vi "Main_SAIDD_v1.1.vi"() -> ()   [LabVIEW 2018]
uses:
  <extravilib>/ChannelInstances/Tag-dbl/Read With Abort.vi
  <extravilib>/ChannelInstances/Tag-bool/Read With Abort.vi
  <extravilib>/ChannelInstances/Tag-u16[State 0 - Default,State 1 - Go down,State 2 - Go up,State 3 - Triangle Wobble]/Read With Abort.vi
  <extravilib>/ChannelInstances/Tag-dbl/Write With Abort.vi
  <extravilib>/ChannelInstances/Tag-bool/Write With Abort.vi
  <extravilib>/ChannelInstances/Tag-u16[State 0 - Default,State 1 - Go down,State 2 - Go up,State 3 - Triangle Wobble]/Write With Abort.vi
  <vilib>/myRIO/Common/Instrument Driver Framework/myRIO v1.0/UART/vis/myRIO v1.0 Close UART.vi
  <vilib>/Utility/error.llb/Error Cluster From Error Code.vi
  <vilib>/myRIO/Common/Instrument Driver Framework/myRIO v1.0/PWM/vis/myRIO v1.0 Write PWM.vi
  <vilib>/myRIO/Common/Instrument Driver Framework/myRIO v1.0/DIO/vis/myRIO v1.0 Write DIO.vi
  <extravilib>/ChannelInstances/Tag-dbl/Instantiate.vi
  <extravilib>/ChannelInstances/Tag-bool/Instantiate.vi
  <extravilib>/ChannelInstances/Tag-u16[State 0 - Default,State 1 - Go down,State 2 - Go up,State 3 - Triangle Wobble]/Instantiate.vi
  <extravilib>/ChannelInstances/Tag-dbl/EndpointRead.vi
  <extravilib>/ChannelInstances/Tag-bool/EndpointRead.vi
  <extravilib>/ChannelInstances/Tag-u16[State 0 - Default,State 1 - Go down,State 2 - Go up,State 3 - Triangle Wobble]/EndpointRead.vi
  <extravilib>/ChannelInstances/Tag-dbl/Endpoint.vi
  <extravilib>/ChannelInstances/Tag-bool/Endpoint.vi
  <extravilib>/ChannelInstances/Tag-u16[State 0 - Default,State 1 - Go down,State 2 - Go up,State 3 - Triangle Wobble]/Endpoint.vi
  <vilib>/myRIO/Common/Instrument Driver Framework/Utilities/vis/FPGA Ref Manager.vi
  <vilib>/myRIO/Common/Instrument Driver Framework/myRIO v1.0/myRIO v1.0 Reset FPGA.vi
  <vilib>/myRIO/Common/Instrument Driver Framework/myRIO v1.0/IRQ/vis/myRIO v1.0 IRQ Info FGV.vi
  <vilib>/myRIO/Common/Instrument Driver Framework/myRIO v1.0/IRQ/vis/myRIO v1.0 Timer IRQ Info FGV.vi
  <vilib>/myRIO/Common/Instrument Driver Framework/myRIO v1.0/IRQ/vis/myRIO v1.0 ISR Agent.vi
  <extravilib>/ChannelInstances/Tag-bool.lvlib
  <vilib>/myRIO/Instrument Drivers/Onboard IO/DIO/DIO.lvlib
  <vilib>/myRIO/Instrument Drivers/Onboard IO/PWM/PWM.lvlib
  <vilib>/myRIO/Instrument Drivers/Utilities/Utilities.lvlib
  <extravilib>/ChannelInstances/Tag-u16[State 0 - Default,State 1 - Go down,State 2 - Go up,State 3 - Triangle Wobble].lvlib
  <extravilib>/ChannelInstances/Tag-dbl.lvlib
panel:
  in  "Tab Control":enum32{"Control", "Test"}(tab)
  in  "Tilt Radius":dbl=0.005 format="%#_13g"
  in  "Cutoff \nFrequency":dbl=900.0
  out "Drill Battery Capacity (%)":dbl(knob) scale=0.0..100.0
  out "Ammeter measurement":dbl(graph)
  in  "Wobble Iterations":i32(knob)=800 scale=500.0..1000.0
  out "Tilt Alarm!":bool
  in  "Stepper \n Frequency":T1(slide)={"Numeric"=120.0, "Numeric"=200.0, "Numeric"=400.0} caption="Stepper Frequency                   Min              Default        Max" scale=100.0..500.0
  in  "Drill Resistance Threshold        Slow            Lower          Upper":T1(slide)={"Numeric"=2750.0, "Numeric"=3025.0, "Numeric"=3100.0} scale=2500.0..3250.0
  out "error out":errorcluster
  in  "Stop":bool
  in  "Enable Triangle Wobble":bool=TRUE
  out "Duty Cycle":dbl
  in  "Drill - Frequency [Hz]":dbl=200.0
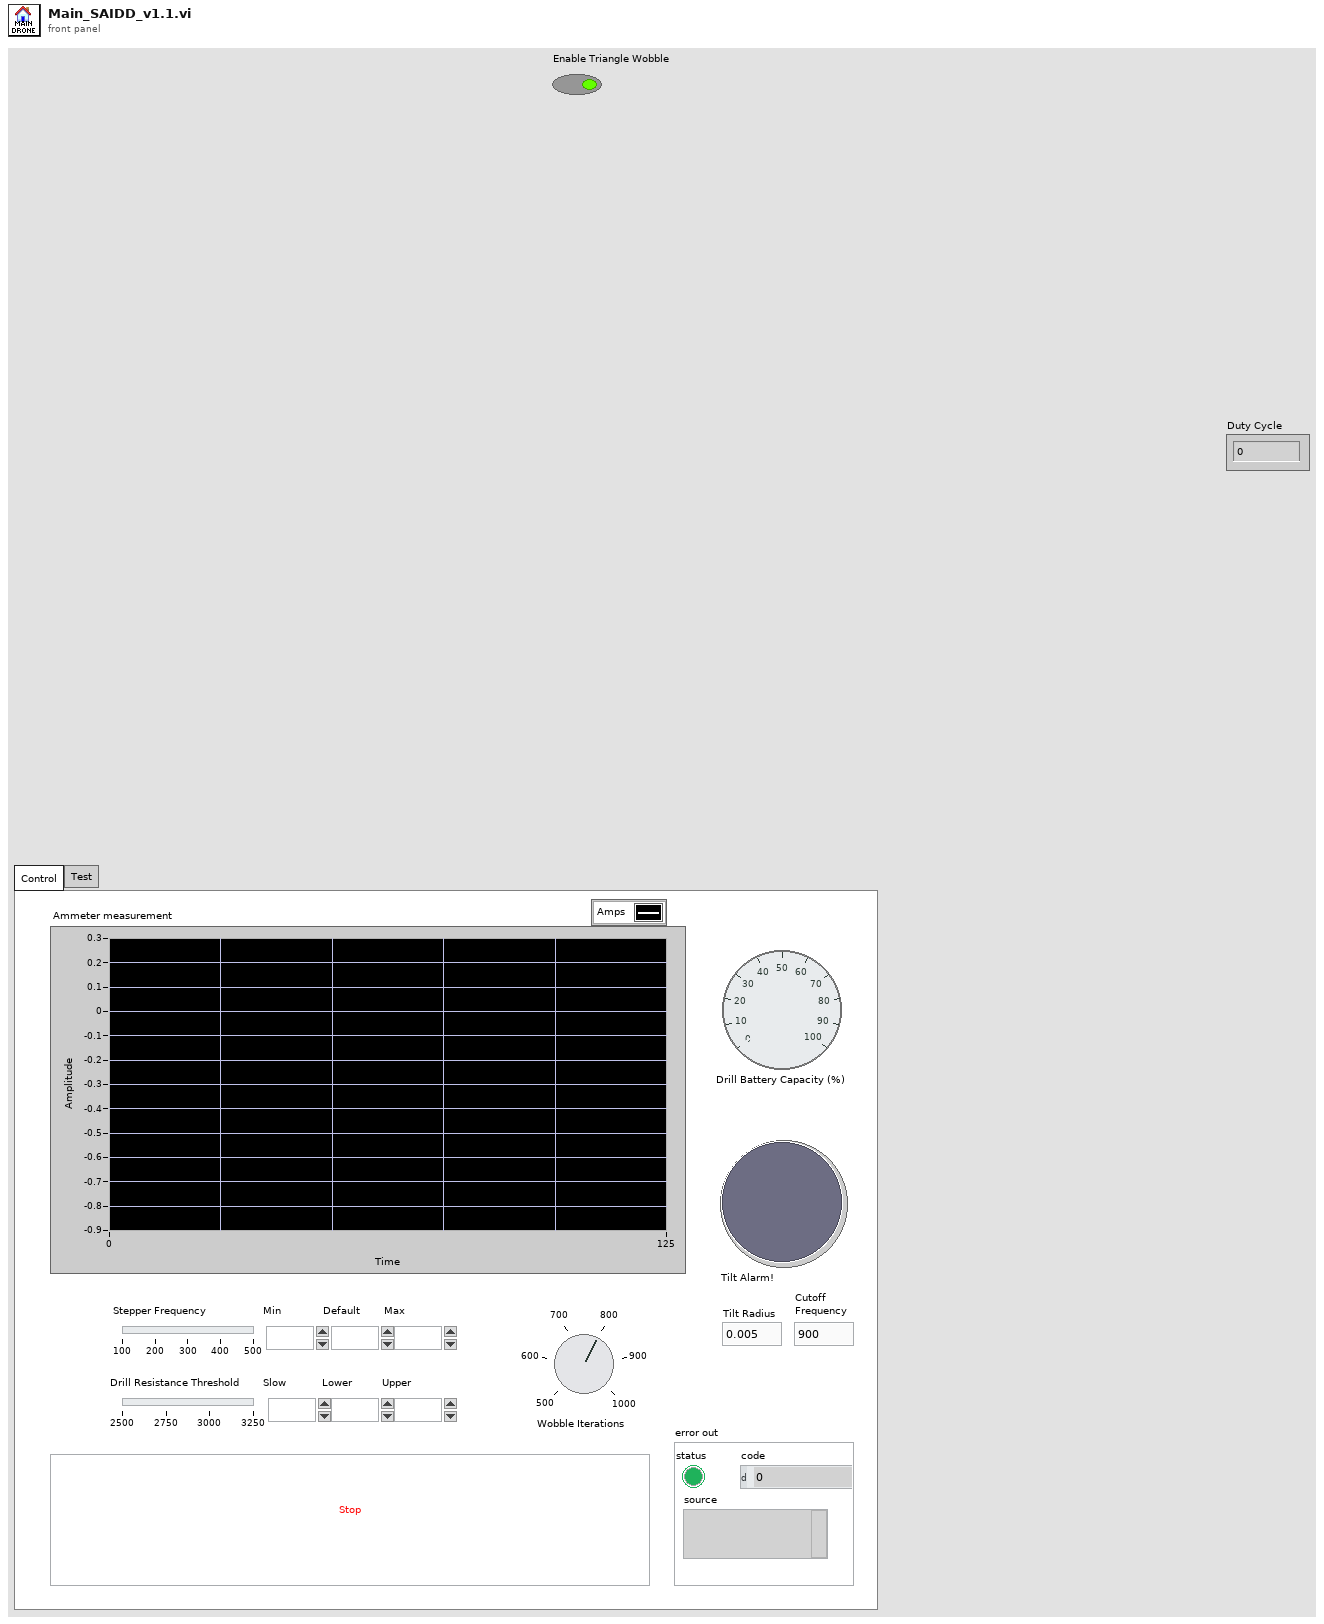
[diagram p1: front panel]
types:
  T1 = cluster{"Numeric":dbl, "Numeric":dbl, "Numeric":dbl}
  T2 = enum16{"State 0 - Default", "State 1 - Go down", "State 2 - Go up", "State 3 - Triangle Wobble"}
  T3 = typedef "DIO.lvlib/DIO Reference.ctl" = cluster{"myRIO Reference":T4, "DIO Channels List":T8}
  T4 = typedef "myRIO Generic Hardware Reference.ctl" = cluster{"myRIO Model":T5, "myRIO Hardware Reference":T6}
  T5 = typedef "Hardware Version Enum.ctl" = enum16{"Unknown", "myRIO-1900", "myRIO-1950", "roboRIO", "NI ELVIS RIO CM", "ELVIS III"}
  T6 = typedef "myRIO v1.0 Reference.ctl" = cluster{"Generic FPGA Reference":T7, "Allow multiple opens":bool}
  T7 = typedef "Generic FPGA Reference.ctl" = refnum<k20>
  T8 = typedef "DIO Channels List.ctl" = T9[]
  T9 = typedef "DIO Channels Enum.ctl" = enum16{"Not Connected", "C/DIO0", "C/DIO1", "C/DIO2", "C/DIO3", "C/DIO4", "C/DIO5", "C/DIO6", "C/DIO7", "A/DIO0", "A/DIO1", "A/DIO2", "A/DIO3", "A/DIO4", "A/DIO5", "A/DIO6", "A/DIO7", "A/DIO8", "A/DIO9", "A/DIO10", "A/DIO11", "A/DIO12", "A/DIO13", "A/DIO14", "A/DIO15", "A/DIO16", "A/DIO17", "A/DIO18", "A/DIO19", "B/DIO0", "B/DIO1", "B/DIO2", "B/DIO3", "B/DIO4", "B/DIO5", "B/DIO6", "B/DIO7", "B/DIO8", "B/DIO9", "B/DIO10", "B/DIO11", "B/DIO12", "B/DIO13", "B/DIO14", "B/DIO15", "B/DIO16", "B/DIO17", "B/DIO18", "B/DIO19", "LED0", "LED1", "LED2", "LED3", "Button0", "DIO/DIO0", "DIO/DIO1", "DIO/DIO2", "DIO/DIO3", "DIO/DIO4", "DIO/DIO5", "DIO/DIO6", "DIO/DIO7", "DIO/DIO8", "DIO/DIO9", "SPI/CS0", "SPI/CS1", "SPI/CS2", "SPI/CS3", "LED RADIO (Green)", "LED RADIO (Red)", "LED COMM (Green)", "LED COMM (Red)", "LED MODE (Green)", "LED MODE (Red)"}
  T10 = typedef "PWM.lvlib/PWM Reference.ctl" = cluster{"myRIO Reference":T4, "PWM Channels Enum":T11, "PWM Configuration":T12}
  T11 = typedef "PWM Channels Enum.ctl" = enum16{"Not Connected", "C/PWM0", "C/PWM1", "A/PWM0", "A/PWM1", "A/PWM2", "A/PWM3", "A/PWM4", "A/PWM5", "A/PWM6", "A/PWM7", "A/PWM8", "A/PWM9", "A/PWM10", "A/PWM11", "A/PWM12", "A/PWM13", "A/PWM14", "A/PWM15", "A/PWM16", "A/PWM17", "A/PWM18", "A/PWM19", "B/PWM0", "B/PWM1", "B/PWM2", "B/PWM3", "B/PWM4", "B/PWM5", "B/PWM6", "B/PWM7", "B/PWM8", "B/PWM9", "B/PWM10", "B/PWM11", "B/PWM12", "B/PWM13", "B/PWM14", "B/PWM15", "B/PWM16", "B/PWM17", "B/PWM18", "B/PWM19", "PWM/PWM0", "PWM/PWM1", "PWM/PWM2", "PWM/PWM3", "PWM/PWM4", "PWM/PWM5", "PWM/PWM6", "PWM/PWM7", "PWM/PWM8", "PWM/PWM9"}
  T12 = typedef "PWM.lvlib/PWM Configuration.ctl" = cluster{"Frequency":dbl, "Duty Cycle":dbl}
  T13 = typedef "Accelerometer.lvlib/Accelerometer Reference.ctl" = cluster{"myRIO Reference":T4, "Accelerometer Channels List":T14, "LSB Weight":dbl}
  T14 = typedef "Accelerometer Channels List.ctl" = T15[]
  T15 = typedef "Accelerometer Channels Enum.ctl" = enum16{"Not Connected", "X-Axis", "Y-Axis", "Z-Axis"}
  T16 = typedef "AI.lvlib/AI Reference.ctl" = cluster{"myRIO Reference":T4, "AI Channels List":T17, "AI Scaling Constants List":T19}
  T17 = typedef "AI Channels List.ctl" = T18[]
  T18 = typedef "AI Channels Enum.ctl" = enum16{"Not Connected", "AudioIn/Left", "AudioIn/Right", "C/AI0", "C/AI1", "A/AI0", "A/AI1", "A/AI2", "A/AI3", "A/AI4", "A/AI5", "A/AI6", "A/AI7", "B/AI0", "B/AI1", "B/AI2", "B/AI3", "B/AI4", "B/AI5", "B/AI6", "B/AI7", "AI/AI0", "AI/AI1", "AI/AI2", "AI/AI3", "A/AI0 (DIFF)", "A/AI1 (DIFF)", "A/AI2 (DIFF)", "A/AI3 (DIFF)", "B/AI0 (DIFF)", "B/AI1 (DIFF)", "B/AI2 (DIFF)", "B/AI3 (DIFF)"}
  T19 = typedef "Analog Scaling Constants List.ctl" = T20[]
  T20 = typedef "Analog Scaling Constants.ctl" = cluster{"LSB Weight (Volts)":dbl, "Offset (Volts)":dbl, "Signed?":bool}
  T21 = typedef "SPI.lvlib/SPI Reference.ctl" = cluster{"myRIO Reference":T4, "SPI Channels Enum":T22, "SPI Configuration":T23}
  T22 = typedef "SPI Channels Enum.ctl" = enum16{"Not Connected", "A/SPI", "B/SPI", "SPI/SPI"}
  T23 = typedef "SPI.lvlib/SPI Configuration.ctl" = cluster{"Frequency [Hz]":dbl, "Clock Phase":T24, "Clock Polarity":T25, "Data Direction":T26, "Frame Length":T27}
  T24 = typedef "SPI Clock Phase.ctl" = enum8{"Leading", "Trailing"}
  T25 = typedef "SPI Clock Polarity.ctl" = enum8{"Low", "High"}
  T26 = typedef "SPI Data Direction.ctl" = enum8{"Most significant bit first", "Least significant bit first"}
  T27 = typedef "SPI Frame Length.ctl" = u8
  T28 = cluster{"B/DIO0 - Stepper Direction":T3, "B/DIO1 - Stepper1 Enable":T3, "B/DIO2 - Stepper2 Enable":T3, "B/DIO3 - Stepper3 Enable":T3, "B/DIO4 - Endstop Stepper1 Top":T3, "B/DIO11 - Endstop Stepper1 Bund":T3, "B/DIO12 - Endstop Stepper2 Top":T3, "B/DIO13 - Endstop Stepper2 Bund":T3, "B/DIO14 - Endstop Stepper3 Top":T3, "B/DIO15 - Endstop Stepper3 Bund":T3, "Deleted - A/DIO0 - Cooler":T3, "A/DIO1 - Beacon drop (dio1)":T3, "A/DIO2 - Beacon drop (dio0)":T3, "A/DIO3 - QuickRelease (dio1)":T3, "A/DIO4 - QuickRelease (dio0)":T3, "Deleted - A/DIO11 - LiDAR SPI CS":T3, "B/PWM0 - Stepper":T10, "B/PWM1 - Drill":T10, "Deleted - A/PWM0 - Servo_Roll":T10, "Deleted - A/PWM1 - Servo_Yaw":T10, "Acc. X-axis":T13, "Acc. Y-axis":T13, "B/AI0 - Drone Grounded S1 - F3":T16, "A/AI0 - QuickRelease S4 - F4":T16, "B/AI2 - Beacon Drop S5 - F5":T16, "B/AI3 - Begin drilling S3 - F6":T16, "B/AI1 - Gimbal Seach S8 - F8":T16, "Deleted - A/AI1 - Beacon Wiper":T16, "A/AI2 - QuickRelease Wiper":T16, "A/AI3 - Drill Current":T16, "Deleted - A/SPI - LiDAR":T21, "B/UART - XBee":refnum<visa-resource-name>, "Deleted - A/UART - A3 GPS":refnum<visa-resource-name>, "RIO Flashing LEDs":T3}
  T29 = typedef "Tag-dbl.lvlib/))Channel.ctl" = refnum<queue>
  T30 = typedef "Tag-bool.lvlib/))Channel.ctl" = refnum<queue>
  T31 = typedef "Tag-u16[State 0 - Default,State 1 - Go down,State 2 - Go up,State 3 - Triangle Wobble].lvlib/))Channel.ctl" = refnum<queue>
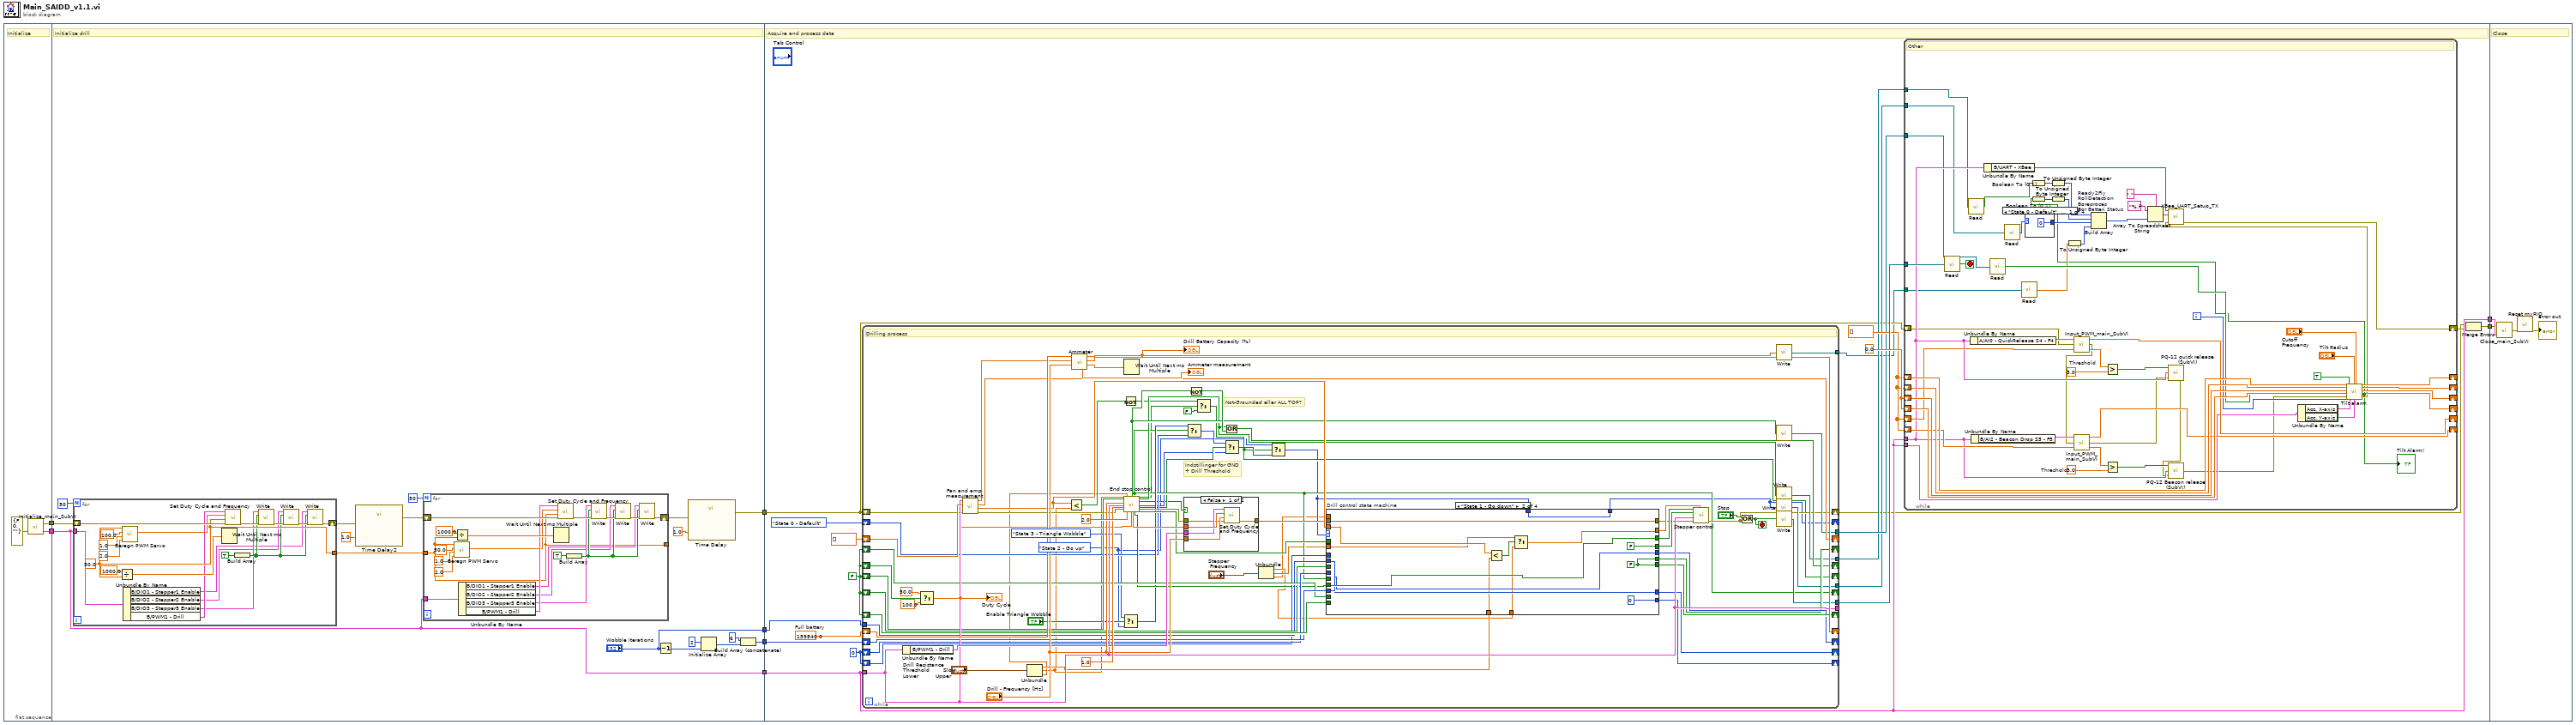
[diagram p0: block diagram]
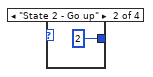
[diagram p2: hidden frame]
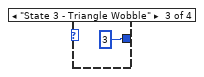
[diagram p3: hidden frame]
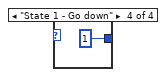
[diagram p4: hidden frame]
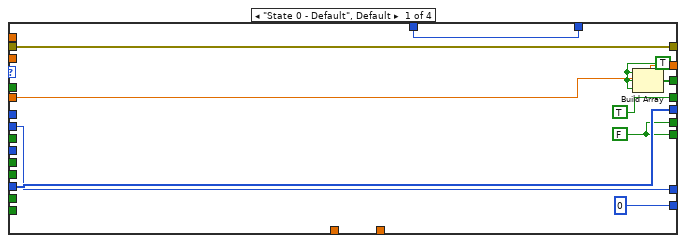
[diagram p6: hidden frame]
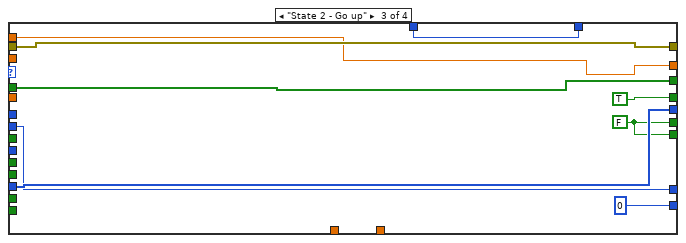
[diagram p7: hidden frame]
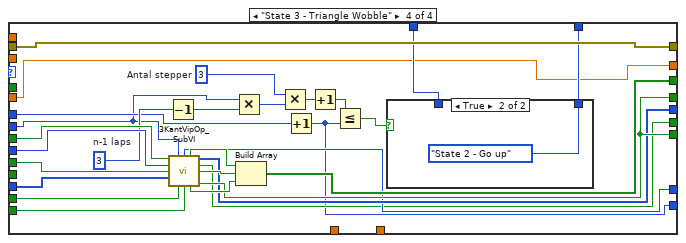
[diagram p8: hidden frame]
diagram:
  n1 = flat-sequence {
    tunnel: [w11] -> w7
    tunnel: [w10] -> w1
    tunnel: w7 -> [w28]
    tunnel: [w28] -> w6
    tunnel: ["Wobble Iterations"] -> w5
    tunnel: [w23] -> w4
    tunnel: [w16] -> w3
    tunnel: w1 -> [w18]
    tunnel: w6 -> [w78]
    tunnel: [w78] -> w8
    tunnel: w5 -> [w81]
    tunnel: w4 -> [w80]
    tunnel: w3 -> [w72]
    tunnel: [w71] -> w2
    tunnel: w8 -> [w299]
    tunnel: w2 -> [w297]
    frame #0 {
      # "Initialize"
      n2 = call "Initialize_main_SubVI.vi"("error in (no error)"=errorcluster {"status"=FALSE, "code"=0, "source"=""}) -> ("output cluster"=w11:T28, "error out"=w10:errorcluster)  [unwired: 1 in]
    }
    frame #1 {
      # "Initialize drill"
      n3 = for {
        N: 50 -> [_]
        tunnel: [w61] -> w21
        shift-right: [w54] -> w19
        shift-left: w18 -> [w63]
        tunnel: w28 -> [w59]
        w61 = 50.0 ("Frequency [Hz]")
        n4 = Divide(x=1000.0, y=w61) -> (x/y=w62:dbl)
        n5 = call "Beregn PWM Servo.vi"("Max (ms puls bredde)"=2.0, "Min (ms puls bredde)"=1.0, "Duty Cycle"=100.0, "Frekvens"=w61) -> ("Output Dutycycle til PWM Servo"=w48:dbl)  [unwired: 7 in]
        n6 = Unbundle By Name(w59) -> ("B/DIO1 - Stepper1 Enable"=w49:T3, "B/DIO2 - Stepper2 Enable"=w50:T3, "B/DIO3 - Stepper3 Enable"=w51:T3, "B/PWM1 - Drill"=w53:T10)
        n7 = Wait Until Next ms Multiple(millisecond multiple=w62) -> ()  [unwired: 1 out]
        n8 = call <vilib>:"Set Duty Cycle and Frequency.vi"("error in (no error)"=w63, "Frequency [Hz]"=w61, "Duty Cycle"=w48, "PWM Ref In"=w53) -> ("error out"=w57:errorcluster)  [unwired: 5 in, 1 out]
        n9 = Build Array(TRUE) -> (w52:bool[])
        n10 = call <extravilib>:"Write.vi"("error in (no error)"=w57, "Values"=w52, "DIO Ref In"=w51) -> ("error out"=w56:errorcluster)  [unwired: 6 in, 1 out]
        n11 = call <extravilib>:"Write.vi"("error in (no error)"=w56, "Values"=w52, "DIO Ref In"=w50) -> ("error out"=w55:errorcluster)  [unwired: 6 in, 1 out]
        n12 = call <extravilib>:"Write.vi"("error in (no error)"=w55, "Values"=w52, "DIO Ref In"=w49) -> ("error out"=w54:errorcluster)  [unwired: 6 in, 1 out]
      }
      n13 = call "Time Delay2"("error in (no error)"=w19, "Delay Time (s)"=1.0) -> ("error out"=w20:errorcluster)  [unwired: 9 in]
      n14 = for {
        N: 50 -> [_]
        tunnel: [w29] -> _
        shift-right: [w36] -> w17
        shift-left: w20 -> [w44]
        tunnel: w28 -> [w41]
        tunnel: w21 -> [w29]
        n15 = call "Beregn PWM Servo.vi"("Max (ms puls bredde)"=2.0, "Min (ms puls bredde)"=1.0, "Duty Cycle"=50.0, "Frekvens"=w29) -> ("Output Dutycycle til PWM Servo"=w30:dbl)  [unwired: 7 in]
        n16 = Divide(x=1000.0, y=w29) -> (x/y=w43:dbl)
        n17 = Unbundle By Name(w41) -> ("B/DIO1 - Stepper1 Enable"=w31:T3, "B/DIO2 - Stepper2 Enable"=w32:T3, "B/DIO3 - Stepper3 Enable"=w33:T3, "B/PWM1 - Drill"=w35:T10)
        n18 = Wait Until Next ms Multiple(millisecond multiple=w43) -> ()  [unwired: 1 out]
        n19 = call <vilib>:"Set Duty Cycle and Frequency.vi"("error in (no error)"=w44, "Frequency [Hz]"=w29, "Duty Cycle"=w30, "PWM Ref In"=w35) -> ("error out"=w39:errorcluster)  [unwired: 5 in, 1 out]
        n20 = Build Array(TRUE) -> (w34:bool[])
        n21 = call <extravilib>:"Write.vi"("error in (no error)"=w39, "Values"=w34, "DIO Ref In"=w33) -> ("error out"=w38:errorcluster)  [unwired: 6 in, 1 out]
        n22 = call <extravilib>:"Write.vi"("error in (no error)"=w38, "Values"=w34, "DIO Ref In"=w32) -> ("error out"=w37:errorcluster)  [unwired: 6 in, 1 out]
        n23 = call <extravilib>:"Write.vi"("error in (no error)"=w37, "Values"=w34, "DIO Ref In"=w31) -> ("error out"=w36:errorcluster)  [unwired: 6 in, 1 out]
      }
      n24 = Decrement(x="Wobble Iterations") -> (x-1=w27:i32)
      n25 = call "Time Delay"("error in (no error)"=w17, "Delay Time (s)"=1.0) -> ("error out"=w16:errorcluster)  [unwired: 9 in]
      n26 = Initialize Array(2, w27) -> (w26:i32[])
      n27 = Build Array (concatenate)(6, w26) -> (w23:i32[])
    }
    frame #2 {
      w82 = 0.0 ("X-Stored-Shift-out")
      w83 = 0 ("Loops shift out")
      w79 = FALSE ("t")
      w85 = 159840.0  # Full battery
      w76 = dbl[] [] ("X-Array-Shift-out")
      # "Acquire and process data"
      n28 = while {
        shift-right: [w175] -> w69
        shift-left: w72 -> [w213]
        shift-right: [w192] -> _
        shift-left: dbl[] [] -> [w224]
        shift-right: [w220] -> _
        shift-left: w85 -> [w221]
        tunnel: w78 -> [w218]
        tunnel: [w218] -> _
        shift-right: [w162] -> _
        shift-left: w79 -> [w214]
        shift-right: [w188] -> _
        shift-left: w79 -> [w211]
        shift-right: [w209] -> _
        shift-left: w79 -> [w208]
        shift-right: [w207] -> _
        shift-left: w80 -> [w206]
        tunnel: w81 -> [w200]
        shift-right: [w204] -> _
        shift-left: w83 -> [w205]
        shift-right: [w203] -> _
        shift-left: w79 -> [w202]
        shift-right: [w173] -> _
        shift-left: w79 -> [w201]
        shift-right: [w198] -> _
        shift-left: w83 -> [w199]
        tunnel: [w185] -> w77
        tunnel: [w183] -> w75
        tunnel: [w182] -> w74
        tunnel: [w180] -> w73
        shift-right: [w157] -> _
        shift-left: T2."State 0 - Default" ("Enum") -> [w172]
        tunnel: [w159] -> w67
        stop <- w186 stop-if-true
        w149 = T2."State 2 - Go up" ("Enum")
        # "Not-Grounded eller ALL TOP?"
        # "Indstillinger for GND \n+ Drill Threshold"
        # "Drilling process"
        n29 = Unbundle By Name(w218) -> ("B/PWM1 - Drill"=w219:T10)
        n30 = Select(t=50.0, s=w211, f=100.0 ("upper limit")) -> (s? t:f=w190:dbl)
        "Duty Cycle" <- w190
        n31 = call "Fan and amp measurement.vi"("error in (no error)"=w213, "Array in"=w224, "output cluster"=w218) -> ("error out"=w179:errorcluster, "Mean out"=w191:dbl, "Array out"=w192:dbl[], "dbl Scaled Value"=w216:dbl)  [unwired: 5 in]
        n32 = Unbundle("Drill Resistance Threshold        Slow            Lower          Upper") -> ("Numeric"=w153:dbl, "Numeric"=w150:dbl, "Numeric"=w152:dbl)
        n33 = Less?(x=w191, y=w150) -> (x < y?=w161:bool)
        n34 = call "Ammeter.vi"("Bor - Frequency [Hz]"="Drill - Frequency [Hz]", "Måling ammeter"=w216, "Sum batteri shift in"=w221) -> ("Wait ud"=w215:dbl, "Sum batteri shift ud"=w220:dbl, "Batteri tilbage (%)"=w160:dbl, "Målt ampere"=→"Ammeter measurement":dbl)  [unwired: 5 in]
        "Drill Battery Capacity (%)" <- w160
        n35 = Not(x=w161) -> (.not. x?=w164:bool)
        n36 = Select(t=T2."State 3 - Triangle Wobble" ("Enum"), s="Enable Triangle Wobble", f=w149) -> (s? t:f=w174:T2)
        n37 = Wait Until Next ms Multiple(millisecond multiple=w215) -> ()  [unwired: 1 out]
        n38 = call "End stop control.vi"("Threshold Lower"=w150, "t"=w214, "Bor - Frequency [Hz]"="Drill - Frequency [Hz]", "output cluster"=w218, "Min (ms puls bredde)"=1.0, "error in (no error)"=w179, "Threshold Upper"=w152, "Max (ms puls bredde)"=2.0, "Bor - Duty Cycle"=w190) -> ("Grounded?"=w184:bool, "Output Dutycycle \nPWM"=w223:dbl, "ALL BOTTOM"=w173:bool, "Bottom Array"=w195:bool[], "Within Drill limits?"=w165:bool, "ALL TOP"=w181:bool, "Move Only?"=w151:bool, "Movement Output"=w168:T2, "HOLD"=w171:bool, "error out"=w178:errorcluster, "Top Array"=w194:bool[])  [unwired: 8 in]
        n39 = case shown="False" w151 {
          tunnel: w223 -> [w231 _]
          tunnel: "Drill - Frequency [Hz]" -> [w230 _]
          tunnel: w219 -> [w229 _]
          tunnel: w178 -> [w228 w232]
          tunnel: [w227 w232] -> w177
          frame False {
            n40 = call <vilib>:"Set Duty Cycle and Frequency.vi"("error in (no error)"=w228, "Frequency [Hz]"=w230, "Duty Cycle"=w231, "PWM Ref In"=w229) -> ("error out"=w227:errorcluster)  [unwired: 5 in, 1 out]
          }
          frame True {
          }
        }
        n41 = Select(t=w174, s=w173, f=w172) -> (s? t:f=w170:T2)
        n42 = Not(x=w184) -> (.not. x?=w187:bool)
        n43 = Select(t=w164, s=w165, f=FALSE) -> (s? t:f=w162:bool)
        n44 = Or(x=w181, y=w187) -> (x .or. y?=w188:bool)
        n45 = Select(t=w170, s=w171, f=w168) -> (s? t:f=w169:T2)
        n46 = Unbundle("Stepper \n Frequency") -> ("Numeric"=w148:dbl, "Numeric"=w155:dbl, "Numeric"=w147:dbl)
        n47 = Select(t=w149, s=w162, f=w169) -> (s? t:f=w158:T2)
        n48 = case "Drill control state machine" shown="\"State 1 - Go down\"" w158 {
          tunnel: [w240 w256 w265 w289] -> w193
          tunnel: w195 -> [_ w256 _ _]
          tunnel: w194 -> [_ _ w265 _]
          tunnel: [TRUE FALSE TRUE w288] -> w217
          tunnel: w177 -> [w239 w254 w263 w293]
          tunnel: [w239 w254 w263 w293] -> w176
          tunnel: [w233 w252 w257 w266] -> w212
          tunnel: w191 -> [_ w251 _ _]
          tunnel: [w236 w248 w260 w288] -> w209
          tunnel: w208 -> [_ _ _ w287]
          tunnel: [w238 w250 w262 w286] -> w207
          tunnel: w206 -> [w238 w250 w262 w285]
          tunnel: w200 -> [w237 w249 w261 w275]
          tunnel: w205 -> [_ _ _ w284]
          tunnel: [w237 w249 w261 w283] -> w204
          tunnel: [w236 w248 w260 w282] -> w203
          tunnel: w202 -> [_ _ _ w281]
          tunnel: w201 -> [_ _ _ w280]
          tunnel: w173 -> [_ _ _ w278]
          tunnel: w199 -> [_ _ _ w277]
          tunnel: [0 0 0 w272] -> w198
          tunnel: w158 -> [w234 w246 w258 w268]
          tunnel: [w234 w246 w258 w267] -> w157
          tunnel: w155 -> [w233 w245 _ w266]
          tunnel: w147 -> [_ _ w257 _]
          tunnel: w148 -> [_ w244 _ _]
          tunnel: w153 -> [_ w243 _ _]
          frame "State 0 - Default", Default {
            w236 = FALSE
            w241 = TRUE
            n49 = Build Array(w241, w241, w241) -> (w240:bool[])
          }
          frame "State 1 - Go down" {
            w248 = FALSE
            n50 = Less?(x=w251, y=w243) -> (x < y?=w253:bool)
            n51 = Select(t=w245, s=w253, f=w244) -> (s? t:f=w252:dbl)
          }
          frame "State 2 - Go up" {
            w260 = FALSE
          }
          frame "State 3 - Triangle Wobble" {
            w273 = 3  # Antal stepper
            w279 = 3  # n-1 laps
            n52 = Decrement(x=w279) -> (x-1=w276:i32)
            n53 = call "3KantVipOp_SubVI.vi"("Shift 1 in"=w280, "Antal iterationer pr. stepper"=w275, "Loops shift in"=w284, "BUND!"=w278, "Index step array shift in"=w285, "Shift 2 in"=w281, "Shift 3 in"=w287) -> ("Loops shift out"=w283:i32, "Enable 1"=w290:bool, "Index step array shift ud"=w286:i32[], "Shift 2 ud"=w282:bool, "Enable 2"=w291:bool, "Enable 3"=w292:bool, "Direction"=w288:bool)  [unwired: 1 in, 1 out]
            n54 = Multiply(x=w275, y=w276) -> (x*y=w274:i32)
            n55 = Build Array(w290, w291, w292) -> (w289:bool[])
            n56 = Multiply(x=w273, y=w274) -> (x*y=w270:i32)
            n57 = Increment(x=w277) -> (x+1=w272:i32)
            n58 = Increment(x=w270) -> (x+1=w269:i32)
            n59 = Less Or Equal?(x=w269, y=w272) -> (x <= y?=w271:bool)
            n60 = case shown="True" w271 {
              tunnel: w268 -> [w294 _]
              tunnel: [w294 T2."State 2 - Go up" ("Enum")] -> w267
              frame False {
              }
              frame True {
              }
            }
          }
        }
        n61 = call "Stepper control.vi"("Stepper frekvens"=w212, "error in (no error)"=w176, "output cluster"=w218, "Direction shift ud"=w217, "Array"=w193) -> ("error out"=w175:errorcluster)  [unwired: 6 in]
        n62 = Or(x="Stop", y=w175) -> (x .or. y?=w186:bool)
        n63 = call <extravilib>:"Write.vi"("element"=w160) -> ("channel"=w159:T29)  [unwired: 1 out]
        n64 = call <extravilib>:"Write.vi"("element"=w184) -> ("channel"=w183:T30)  [unwired: 1 out]
        n65 = call <extravilib>:"Write.vi"("element"=w181) -> ("channel"=w180:T30)  [unwired: 1 out]
        n66 = call <extravilib>:"Write.vi"("element"=w157) -> ("channel"=w182:T31)  [unwired: 1 out]
        n67 = call <extravilib>:"Write.vi"("element"=w186) -> ("channel"=w185:T30)  [unwired: 1 out]
      }
      n68 = while {
        shift-right: [w137] -> _
        shift-left: w76 -> [w142]
        shift-right: [w136] -> _
        shift-left: w76 -> [w141]
        shift-right: [w135] -> _
        shift-left: w82 -> [w140]
        shift-right: [w134] -> _
        shift-left: w82 -> [w139]
        tunnel: w77 -> [w133]
        tunnel: w78 -> [w126]
        tunnel: w78 -> [w127]
        shift-right: [w131] -> _
        shift-left: w76 -> [w130]
        shift-right: [w129] -> _
        shift-left: w76 -> [w128]
        tunnel: w75 -> [w125]
        tunnel: w74 -> [w123]
        tunnel: w73 -> [w122]
        shift-right: [w93] -> w70
        shift-left: w72 -> [w94]
        tunnel: w67 -> [w92]
        i -> [w138]
        stop <- w132 stop-if-true
        w115 = 3.0  # Threshold
        w121 = 3.0  # Threshold
        # "Other"
        n69 = call <extravilib>:"Read.vi"("channel"=w133) -> ("element"=w132:bool)  [unwired: 1 in, 1 out]
        n70 = call <extravilib>:"Read.vi"("channel"=w122) -> ("element"=w96:bool)  [unwired: 1 in, 1 out]
        n71 = Unbundle By Name(w127) -> ("A/AI0 - QuickRelease S4 - F4"=w117:T16)
        n72 = Unbundle By Name(w127) -> ("B/AI2 - Beacon Drop S5 - F5"=w119:T16)
        n73 = Unbundle By Name(w127) -> ("B/UART - XBee"=w107:refnum<visa-resource-name>)
        n74 = call <extravilib>:"Read.vi"("channel"=w125) -> ("element"=w124:bool)  [unwired: 1 in, 1 out]
        n75 = call <extravilib>:"Read.vi"("channel"=w123) -> ("element"=w97:T2)  [unwired: 1 in, 1 out]
        n76 = call <extravilib>:"Read.vi"("channel"=w92) -> ("element"=w90:dbl)  [unwired: 1 in, 1 out]
        n77 = case shown="\"State 0 - Default\", Default" w97 {
          tunnel: [u8 0 u8 2 u8 3 u8 1] -> w102
          frame "State 0 - Default", Default {
          }
          frame "State 2 - Go up" {
          }
          frame "State 3 - Triangle Wobble" {
          }
          frame "State 1 - Go down" {
          }
        }
        n78 = Boolean To (0,1)(Boolean=w96) -> (0, 1=w101:i16)
        n79 = To Unsigned Byte Integer(number=w101) -> (unsigned 8bit integer=w100:u8)
        n80 = To Unsigned Byte Integer(number=w90) -> (unsigned 8bit integer=w91:u8)
        n81 = call "Input_PWM_main_SubVI.vi"("Shift in"=w130, "error in (no error)"=w94, "AI Ref In"=w117) -> ("Value out"=w116:dbl, "error out"=w113:errorcluster, "Shift out"=w131:dbl[])
        n82 = call "Input_PWM_main_SubVI.vi"("Shift in"=w128, "error in (no error)"=w113, "AI Ref In"=w119) -> ("Value out"=w120:dbl, "error out"=w89:errorcluster, "Shift out"=w129:dbl[])
        n83 = Greater?(x=w116, y=w115) -> (0:w114:bool)
        n84 = Greater?(x=w120, y=w121) -> (0:w118:bool)
        n85 = call "PQ-12 quick release (SubVI).vi"("error in (no error)"=w89, "output cluster"=w127, "Extend / Retract [F/T]"=w114) -> ("error out"=w88:errorcluster)
        n86 = call "PQ-12 Beacon release (SubVI).vi"("error in (no error)"=w88, "output cluster"=w127, "Extend / Retract [T/F]"=w118) -> ("error out"=w87:errorcluster)
        n87 = Unbundle By Name(w126) -> ("Acc. X-axis"=w111:T13, "Acc. Y-axis"=w112:T13)
        n88 = call "Tilt alarm.vi"("X-Array-Shift-in"=w142, "Y-Array-Shift-in"=w141, "X-Stored-Shift-in"=w140, "Y-Stored-Shift-in"=w139, "Grounded?"=w124, "error in (no error)"=w87, "Iterations"=w138, "Filter?"=TRUE, "Accelerometer Ref X in"=w111, "Radius"="Tilt Radius", "Accelerometer Ref Y In"=w112, "high cutoff freq: fh"="Cutoff \nFrequency") -> ("X-Array-Shift-out"=w137:dbl[], "Y-Array-Shift-out"=w136:dbl[], "X-Stored-Shift-out"=w135:dbl, "Y-Stored-Shift-out"=w134:dbl, "Alarm"=w86:bool, "error out"=w95:errorcluster)  [unwired: 10 in]
        "Tilt Alarm!" <- w86
        n89 = Boolean To (0,1)(Boolean=w86) -> (0, 1=w99:i16)
        n90 = To Unsigned Byte Integer(number=w99) -> (unsigned 8bit integer=w98:u8)
        n91 = Build Array "Ready2Fly\nRollDetection\nBoreproces\nBor Batteri Status"(w100, w98, w102, w91) -> (w103:u8[])
        n92 = Array To Spreadsheet String(delimiter (Tab)=",", array=w103, 3:"%.f" ("format string")) -> (spreadsheet string=w106:string)
        n93 = call "XBee_UART_Setup_TX.vi"("error in (no error)"=w95, "Characters to Write"=w106, "VISA resource name in"=w107) -> ("error out"=w93:errorcluster)  [unwired: 8 in]
      }
      n94 = Merge Errors(w69, w70) -> (w71:errorcluster)
    }
    frame #3 {
      # "Close"
      n95 = call "Close_main_SubVI.vi"("output cluster"=w299, "error in (no error)"=w297) -> ("error out"=w298:errorcluster)
      n96 = call <vilib>:"Reset myRIO.vi"("error in (no error)"=w298) -> ("error out"=→"error out":errorcluster)  [unwired: 10 in]
    }
  }
